vi "RecvData.vi"(0 "ID":i32=10, 1 "类型":u32(ring)=4 items=["PCI5121"=1, "PCI9810"=2, "USBCAN1"=3, "USBCAN2"=4, "PCI9820"=5, "CAN232"=6, "PCI5110"=7, "CANLite(mini)"=8, "ISA9620"=9, "ISA5420"=10, "PC104CAN"=11, "CANET"=17, "DNP9810"=13, "USBCAN-E-U"=20, "USBCAN-2E-U"=21], 2 "设备索引":u32(ring) items=["0", "1", "2", "3", "4", "5", "6", "7", "8", "9", "10", "11", "12", "13", "14", "15", ""], 3 "CAN路数":u32(ring) items=["0", "1"], 5 "start bit":u8=10, 9 "bit len":u8=10, 11 "time out":u32) -> (4 "recv ok?":bool, 6 "Value":u64)   [LabVIEW 2018]
uses:
  ControlCAN/64/ControlCAN.dll
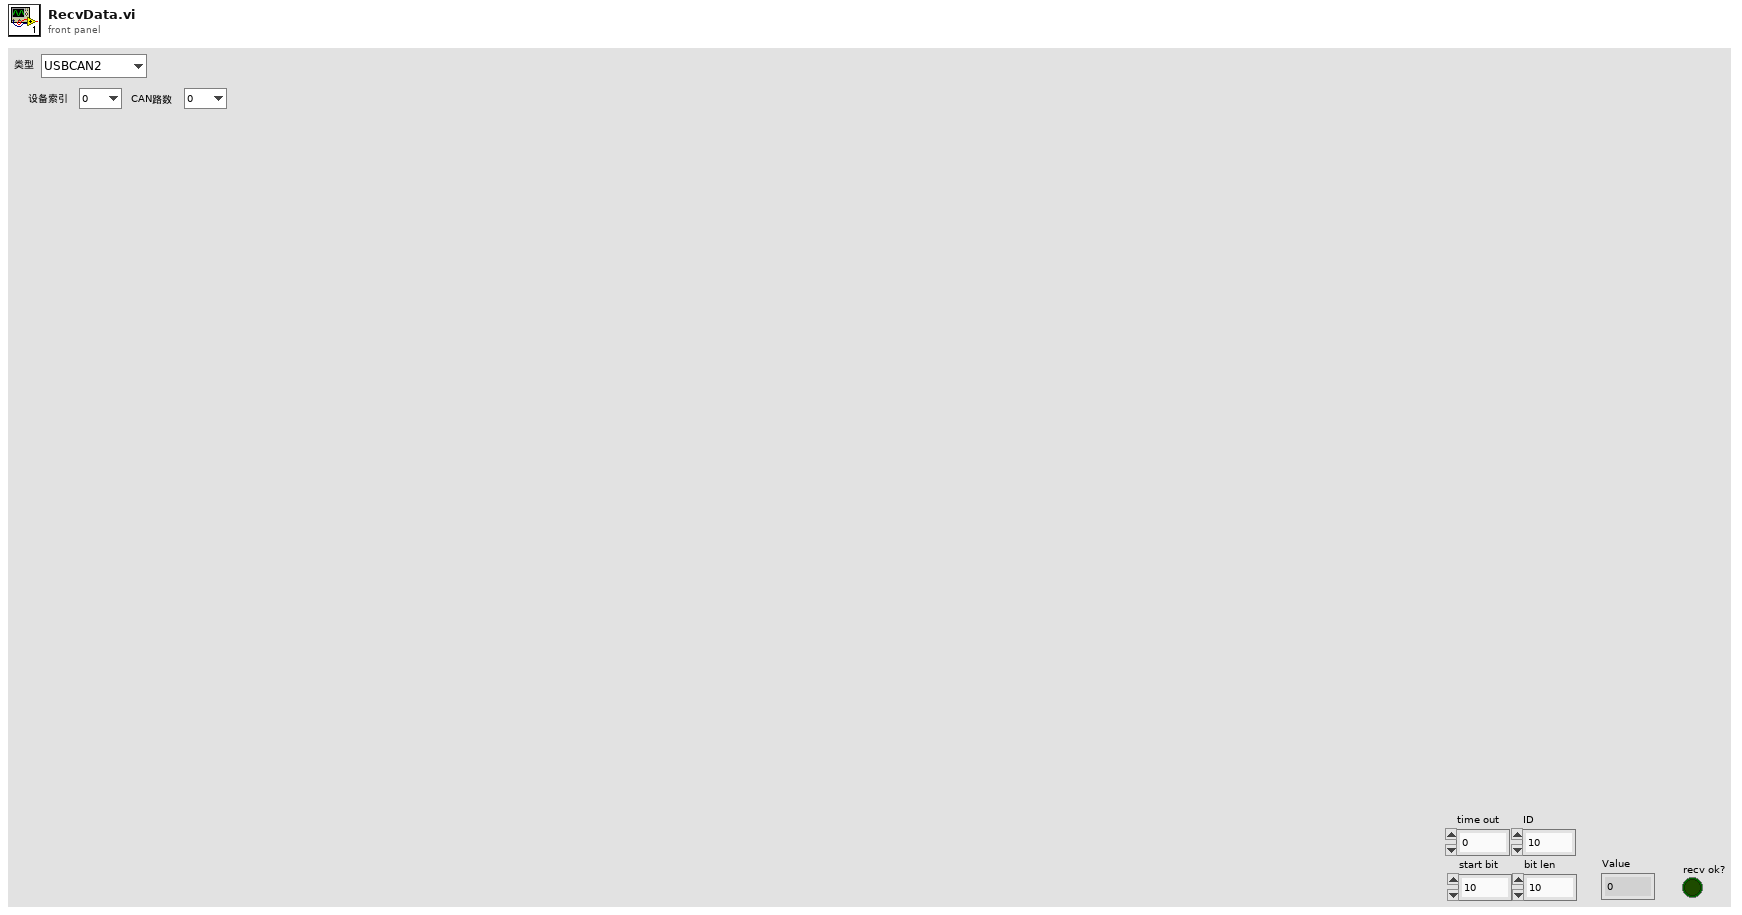
[diagram p1: front panel]
types:
  T1 = cluster{"ID":u32, "TimeStamp":u32, "TimeFlag":u8, "SendType":u8, "RemoteFlag":u8, "ExternFlag":u8, "DataLen":u8, u8, u8, u8, u8, u8, u8, u8, u8, u8, u8, u8}
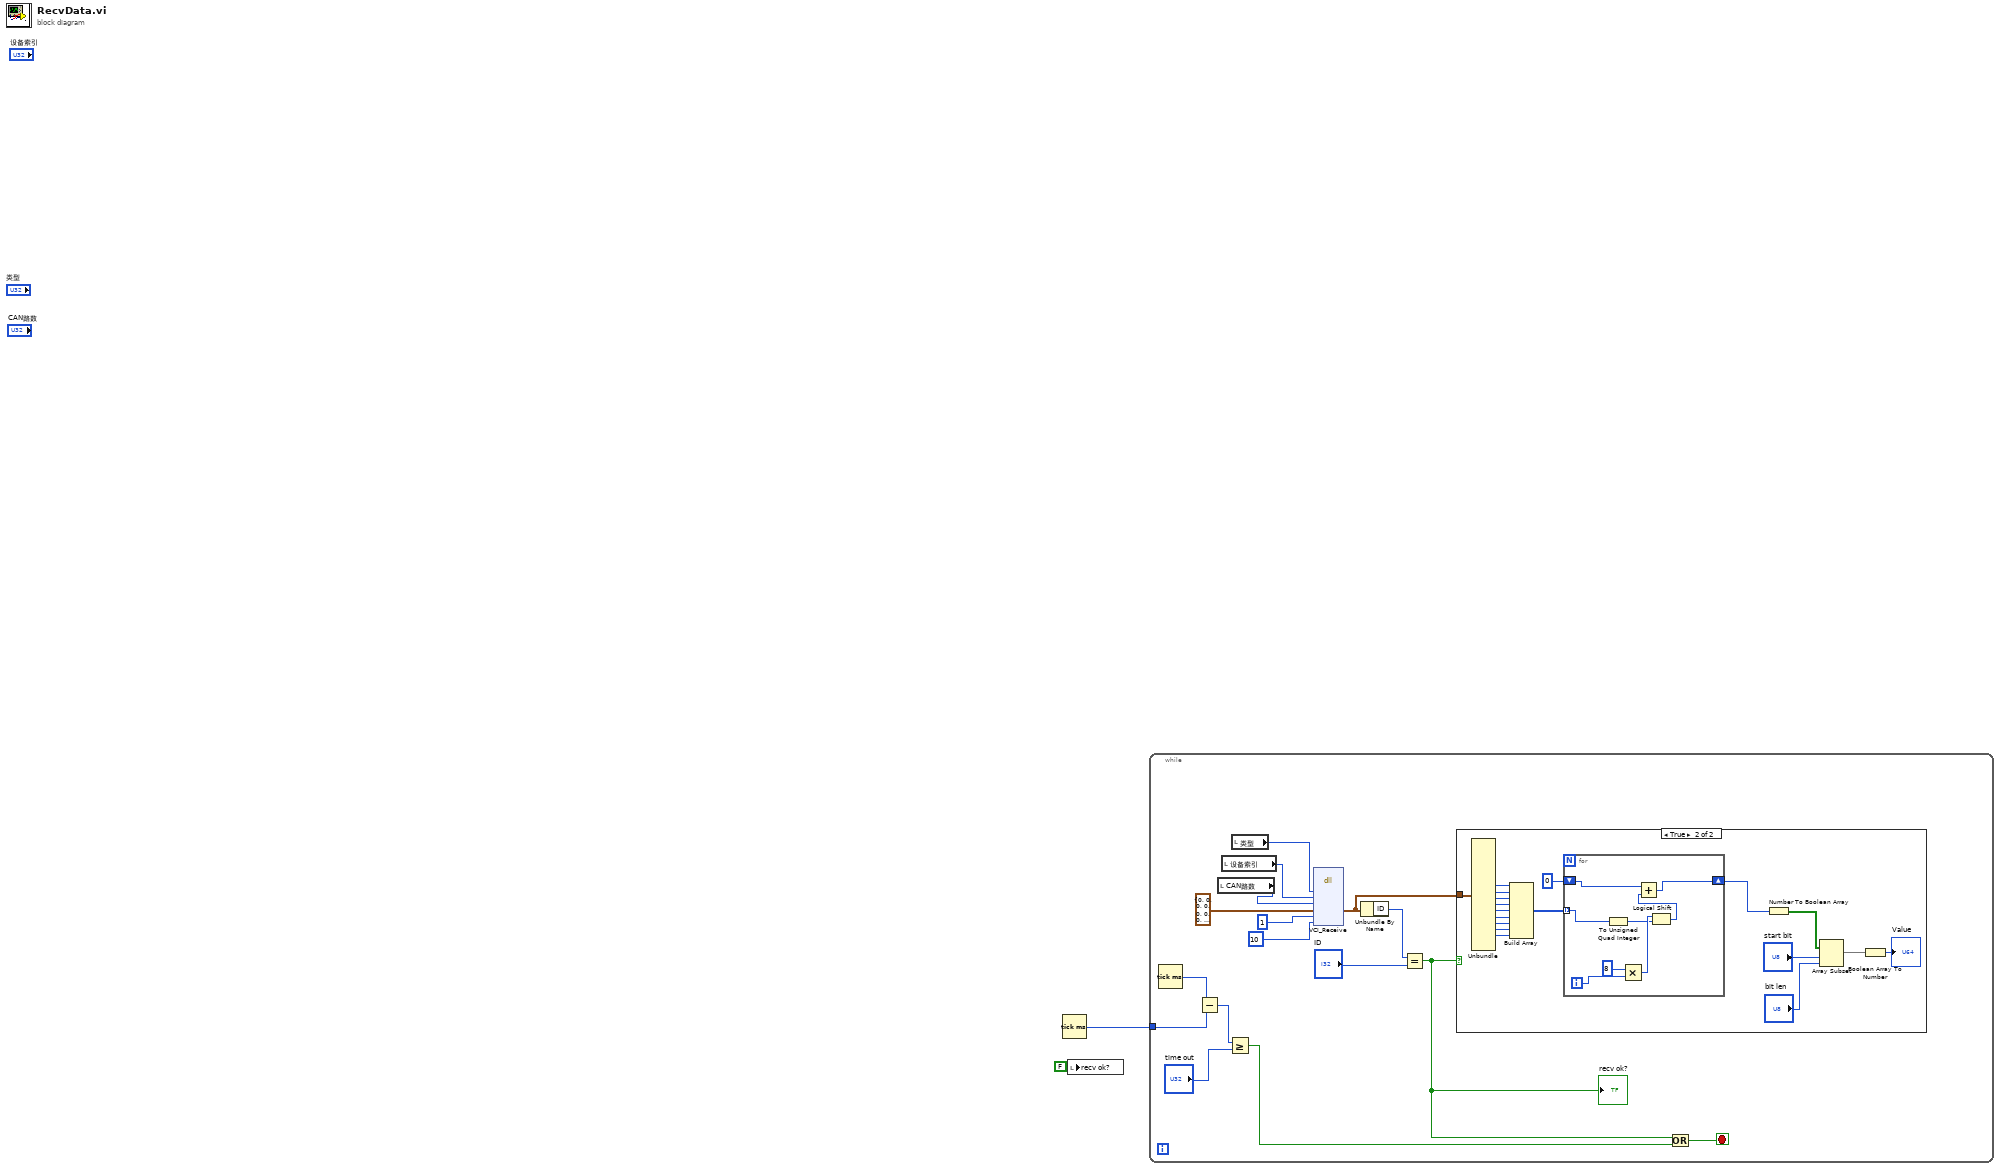
[diagram p0: block diagram]
diagram:
  n1 = Tick Count (ms)() -> (millisecond timer value=w2:u32)
  n2 = local write "recv ok?"(FALSE ("x = y?")) -> ()
  n3 = while {
    tunnel: w2 -> [w11]
    stop <- w4 stop-if-true
    n4 = Tick Count (ms)() -> (millisecond timer value=w12:u32)
    n5 = Subtract(x=w12, y=w11) -> (x-y=w10:u32)
    n6 = local read "CAN路数"() -> (w16:u32)
    n7 = local read "设备索引"() -> (w13:u32)
    n8 = Greater Or Equal?(x=w10, y="time out") -> (x >= y?=w5:bool)
    n9 = local read "类型"() -> (w14:u32)
    n10 = dll-call lib="C:/Users/Administrator/Desktop/AutoTest_TestStand/trunk/AutoTest_TestStand/Driver/ZlgCan/ControlCAN/64/ControlCAN.dll" fn="VCI_Receive"("DeviceType"=w14, "DeviceInd"=w13, "CANInd"=w16, "pReceive"=T1 {"ID"=0, "TimeStamp"=0, "TimeFlag"=0, "SendType"=0, "RemoteFlag"=0, "ExternFlag"=0, "DataLen"=0, 0, 0, 0, 0, 0, 0, 0, 0, 0, 0, 0}, "Len"=u32 1, "WaitTime"=10) -> ("pReceive"=w3:T1)  [unwired: 8 in, 3 out]
    n11 = Unbundle By Name(w3) -> ("ID"=w8:u32)
    n12 = Equal?(x=w8, y="ID") -> (x = y?=w6:bool)
    "recv ok?" <- w6
    n13 = case shown="True" w6 {
      tunnel: w3 -> [_ w36]
      frame False {
      }
      frame True {
        n14 = Unbundle(w36) -> (w35:u8, w34:u8, w33:u8, w32:u8, w31:u8, w30:u8, w29:u8, w28:u8, w27:u8)  [unwired: 9 out]
        n15 = Build Array(w35, w34, w33, w32, w31, w30, w29, w28, w27) -> (w26:u8[])
        n16 = for {
          tunnel: w26 -> [w38] mode=indexing
          shift-right: [w43] -> w24
          shift-left: u64 0 -> [w44]
          i -> [w41]
          n17 = To Unsigned Quad Integer(1:w38) -> (0:w37:u64)
          n18 = Multiply(x=8, y=w41) -> (x*y=w39:i32)
          n19 = Logical Shift(y=w39, x=w37) -> (x << y=w42:u64)
          n20 = Add(x=w44, y=w42) -> (x+y=w43:u64)
        }
        n21 = Number To Boolean Array(number=w24) -> (Boolean array=w23:bool[])
        n22 = Array Subset(array=w23, index="start bit", length="bit len") -> (w20:bool[])
        n23 = Boolean Array To Number(Boolean array=w20) -> (number=→"Value":u32)
      }
    }
    n24 = Or(x=w6, y=w5) -> (x .or. y?=w4:bool)
  }
